vi "Convert_Time_Parameter.vi"(0 "Data":T1 {"Target_Type" items=["10 Bit Address", "7 Bit Address"]; "Selected_Register_Address" format="%x"; "Target_Address" format="%x"}) -> (4 "Converted_Data":T3)   [LabVIEW 2021]
doc: "Used to convert the time parameters"
uses:
  Controls/Time_Parameter.ctl
  Controls/I2C_Data.ctl
  Controls/Customized_Ring.ctl
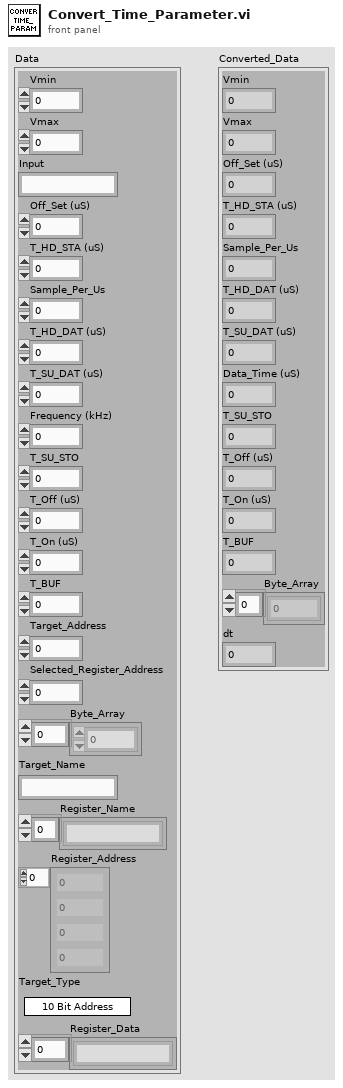
[diagram p1: front panel]
types:
  T1 = typedef "I2C_Data.ctl" = cluster{"Vmin":dbl, "Vmax":dbl, "Input":string, "Off_Set (uS)":dbl, "T_HD_STA (uS)":dbl, "Sample_Per_Us":dbl, "T_HD_DAT (uS)":dbl, "T_SU_DAT (uS)":dbl, "Frequency (kHz)":dbl, "T_SU_STO":dbl, "T_Off (uS)":dbl, "T_On (uS)":dbl, "T_BUF":dbl, "Target_Address":u16, "Selected_Register_Address":u8, "Byte_Array":u8[], "Target_Name":string, "Register_Name":string[], "Register_Address":u8[], "Target_Type":T2, "Register_Data":string[]}
  T2 = typedef "Customized_Ring.ctl" = u16
  T3 = typedef "Time_Parameter.ctl" = cluster{"Vmin":dbl, "Vmax":dbl, "Off_Set (uS)":i32, "T_HD_STA (uS)":i32, "Sample_Per_Us":i32, "T_HD_DAT (uS)":i32, "T_SU_DAT (uS)":i32, "Data_Time (uS)":i32, "T_SU_STO":i32, "T_Off (uS)":i32, "T_On (uS)":i32, "T_BUF":i32, "Byte_Array":u8[], "dt":dbl}
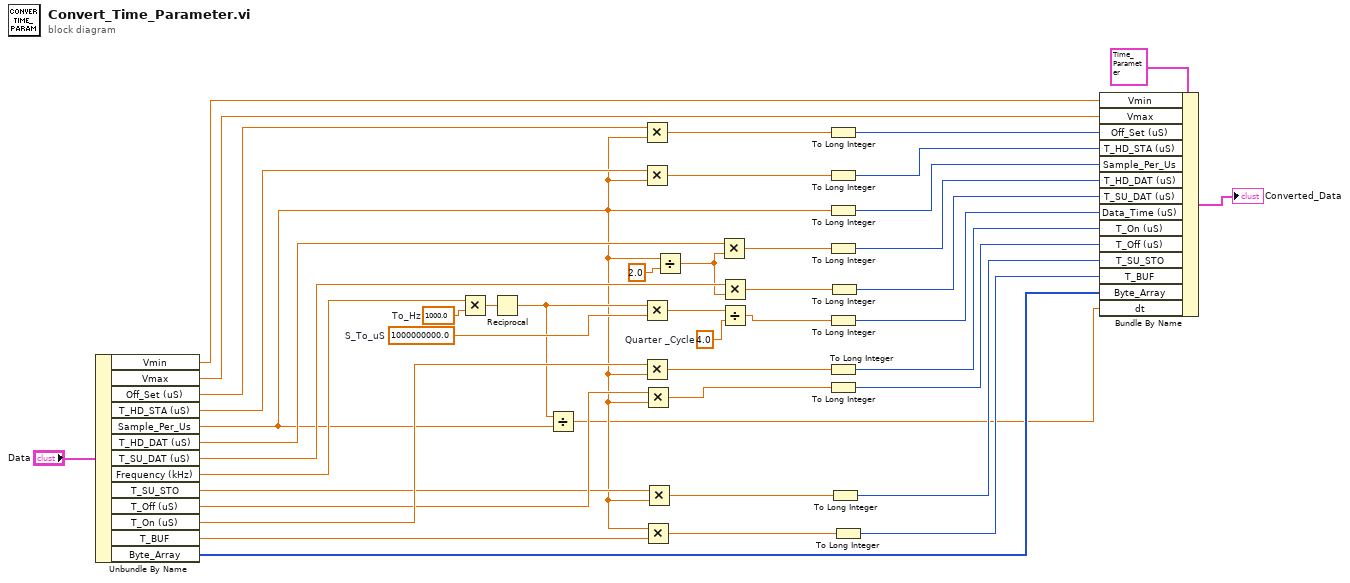
[diagram p0: block diagram]
diagram:
  w14 = 4.0  # Quarter _Cycle
  w10 = 1000.0  # To_Hz
  w16 = 1000000000.0  # S_To_uS
  n1 = Unbundle By Name("Data") -> ("Vmin"=w32:dbl, "Vmax"=w33:dbl, "Off_Set (uS)"=w27:dbl, "T_HD_STA (uS)"=w26:dbl, "Sample_Per_Us"=w2:dbl, "T_HD_DAT (uS)"=w25:dbl, "T_SU_DAT (uS)"=w24:dbl, "Frequency (kHz)"=w4:dbl, "T_SU_STO"=w21:dbl, "T_Off (uS)"=w22:dbl, "T_On (uS)"=w23:dbl, "T_BUF"=w7:dbl, "Byte_Array"=w5:u8[])
  n2 = Multiply(x=w4, y=w10) -> (x*y=w9:dbl)
  n3 = Reciprocal(x=w9) -> (1/x=w3:dbl)
  n4 = Divide(x=w3, y=w2) -> (x/y=w1:dbl)
  n5 = Multiply(x=w27, y=w2) -> (x*y=w11:dbl)
  n6 = Multiply(x=w26, y=w2) -> (x*y=w12:dbl)
  n7 = Multiply(x=w3, y=w16) -> (x*y=w13:dbl)
  n8 = Multiply(x=w23, y=w2) -> (x*y=w30:dbl)
  n9 = Multiply(x=w22, y=w2) -> (x*y=w29:dbl)
  n10 = Multiply(x=w2, y=w7) -> (x*y=w6:dbl)
  n11 = Multiply(x=w21, y=w2) -> (x*y=w17:dbl)
  n12 = Divide(x=w2, y=2.0) -> (x/y=w19:dbl)
  n13 = Multiply(x=w25, y=w19) -> (x*y=w28:dbl)
  n14 = Multiply(x=w24, y=w19) -> (x*y=w15:dbl)
  n15 = Divide(x=w13, y=w14) -> (x/y=w8:dbl)
  n16 = To Long Integer(number=w11) -> (32bit integer=w34:i32)
  n17 = To Long Integer(number=w12) -> (32bit integer=w35:i32)
  n18 = To Long Integer(number=w2) -> (32bit integer=w36:i32)
  n19 = To Long Integer(number=w28) -> (32bit integer=w37:i32)
  n20 = To Long Integer(number=w8) -> (32bit integer=w39:i32)
  n21 = To Long Integer(number=w30) -> (32bit integer=w40:i32)
  n22 = To Long Integer(number=w29) -> (32bit integer=w41:i32)
  n23 = To Long Integer(number=w15) -> (32bit integer=w38:i32)
  n24 = To Long Integer(number=w17) -> (32bit integer=w42:i32)
  n25 = To Long Integer(number=w6) -> (32bit integer=w43:i32)
  n26 = Bundle By Name(cluster=T3 {"Vmin"=0.0, "Vmax"=1.0, "Off_Set (uS)"=0, "T_HD_STA (uS)"=0, "Sample_Per_Us"=0, "T_HD_DAT (uS)"=0, "T_SU_DAT (uS)"=0, "Data_Time (uS)"=0, "T_SU_STO"=0, "T_Off (uS)"=0, "T_On (uS)"=0, "T_BUF"=0, "Byte_Array"=[], "dt"=0.0}, "Vmin"=w32, "Vmax"=w33, "Off_Set (uS)"=w34, "T_HD_STA (uS)"=w35, "Sample_Per_Us"=w36, "T_HD_DAT (uS)"=w37, "T_SU_DAT (uS)"=w38, "Data_Time (uS)"=w39, "T_On (uS)"=w40, "T_Off (uS)"=w41, "T_SU_STO"=w42, "T_BUF"=w43, "Byte_Array"=w5, "dt"=w1) -> (→"Converted_Data":T3)
